vi "NumericPad-Dual.vi"() -> ()   [LabVIEW 2009]
uses:
  <vilib>/NXT/Subs/LVHSConnector.ctl
  <vilib>/NXT/Block Support/NXT_InputPort.ctl
  mindsensors.com LVEE Toolkit/Dual/NumericPad-DM.vi
panel:
  out "Output Cluster":T1={"Key Numeric Value"=49, "Key String Value"="1", "Key match found"=FALSE}
  out "NXT dup":T2={"error"={"status"=FALSE, "code"=0, "source"=""}, "address"="USB0::0x0694::0x0002::001653FF017B::RAW", "NXT #"=0, "Show Error"=TRUE, "Connection"=4} {"Connection" items=["USB", "Bluetooth", "USB then Bluetooth", "Last Connection", "Preference"]}
  in  "Input Port":T3 items=["Port 1", "Port 2", "Port 3", "Port 4"]
  in  "NXT":T2={"error"={"status"=FALSE, "code"=0, "source"=""}, "address"="USB0::0x0694::0x0002::001653FF017B::RAW", "NXT #"=0, "Show Error"=TRUE, "Connection"=4} {"Connection" items=["USB", "Bluetooth", "USB then Bluetooth", "Last Connection", "Preference"]}
  in  "Input Cluster":T4={"Operation"=0, "Wait for (ms):"=1000, "Look for key press:"=49} {"Look for key press:" items=["Key_1"=49, "Key_2"=50, "Key_3"=51, "Key_4"=52, "Key_5"=53, "Key_6"=54, "Key_7"=55, "Key_8"=56, "Key_9"=57, "Key_0"=48, "Key_#"=35, "Key_*"=42]; "Operation" items=["ReadPad", "InitializeSetup"]}
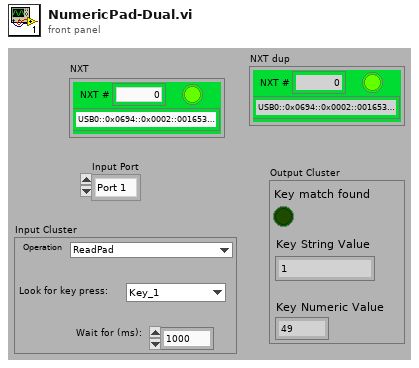
[diagram p1: front panel]
types:
  T1 = cluster{"Key Numeric Value":u8, "Key String Value":string, "Key match found":bool}
  T2 = typedef "LVHSConnector.ctl" = cluster{"error":errorcluster, "address":string, "NXT #":i32, "Show Error":bool, "Connection":u16}
  T3 = typedef "NXT_InputPort.ctl" = u8
  T4 = cluster{"Operation":u8, "Wait for (ms):":i16, "Look for key press:":u8}
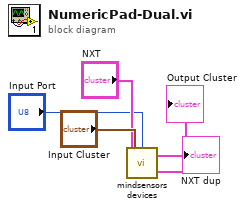
[diagram p0: block diagram]
diagram:
  n1 = call-poly "mindsensors devices.vi"("Input Cluster"="Input Cluster", "NXT"="NXT", "Input Port"="Input Port") -> ("Output Cluster"=→"Output Cluster":T1, "NXT dup"=→"NXT dup":T2)
